vi "datalog.vi"(0 "object in":refnum<class "interface.lvclass">, 1 "data":string, 2 "filename":string="报文记录", 5 "error in (no error)":errorcluster) -> (14 "object out":refnum<class "interface.lvclass">, 19 "error out":errorcluster)   [LabVIEW 2016, in "interface.lvclass"]
uses:
  interface.lvclass
panel:
  out "路径":path
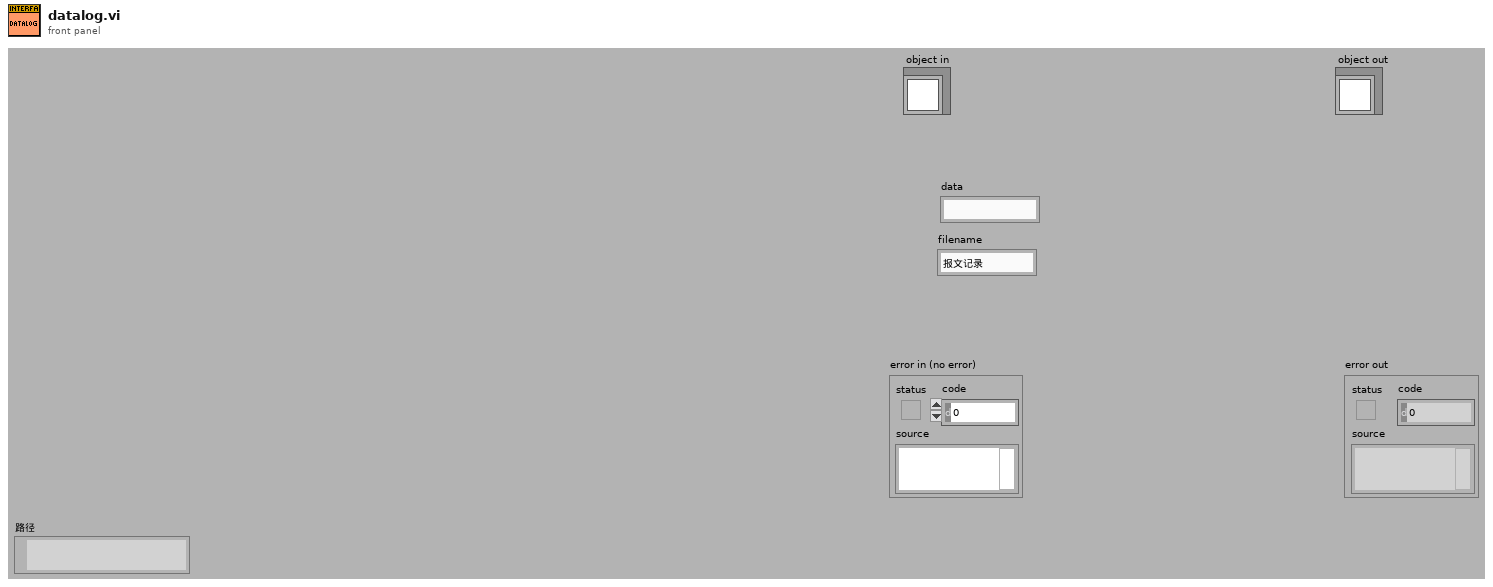
[diagram p1: front panel]
types:
  T1 = enum16{"open", "replace", "create", "open or create", "replace or create", "replace or create with confirmation"}
  T2 = typedef "LVDateTimeRec.ctl" = cluster{"秒数的小数部分":dbl, "秒":i32, "分":i32, "时":i32, "日":i32, "月":i32, "年":i32, "天数（周）":i32, "天数（年）":i32, "DST":i32}
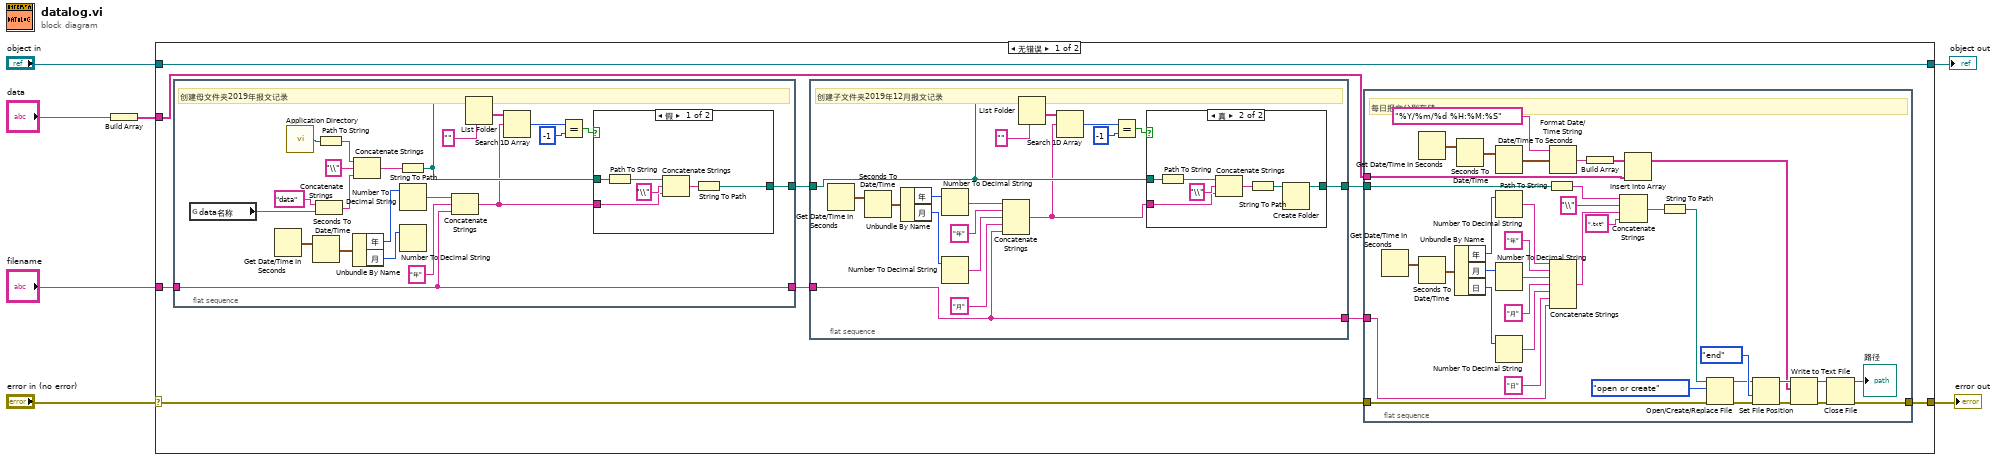
[diagram p0: block diagram]
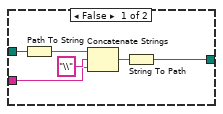
[diagram p2: hidden frame]
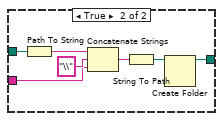
[diagram p3: hidden frame]
diagram:
  n1 = Build Array("data") -> (w1:string[])
  n2 = case shown="无错误" "error in (no error)" {
    selector: "error in (no error)" -> [w8 w121]
    tunnel: [w9 w121] -> w6
    tunnel: [w16 w120] -> w4
    tunnel: "object in" -> [w16 w120]
    tunnel: "filename" -> [w11 _]
    tunnel: w1 -> [w10 _]
    frame No Error {
      n3 = flat-sequence {
        tunnel: [w89] -> w15
        tunnel: [w86] -> w13
        tunnel: w11 -> [w86]
        frame #0 {
          # "创建母文件夹2019年报文记录"
          n4 = global read "断电保存全局.vi" "data名称"() -> (w85:string)
          n5 = Get Date/Time In Seconds() -> (seconds since 1Jan1904=w106:timestamp)
          n6 = call <vilib>:"Application Directory.vi"() -> ("Application Directory"=w94:path)
          n7 = Seconds To Date/Time(time stamp (now)=w106) -> (date time rec=w105:T2)  [unwired: 1 in]
          n8 = Concatenate Strings("data" ("名称或相对路径"), w85) -> (w87:string)
          n9 = Path To String(path=w94) -> (string=w97:string)
          n10 = Unbundle By Name(w105) -> ("年"=w104:i32, "月"=w103:i32)
          n11 = Concatenate Strings(w97, "\\" ("字符串"), w87) -> (w95:string)
          n12 = String To Path(string=w95) -> (path=w93:path)
          n13 = Number To Decimal String(number=w104) -> (decimal integer string=w91:string)  [unwired: 1 in]
          n14 = Number To Decimal String(number=w103) -> ()  [unwired: 1 in, 1 out]
          n15 = Concatenate Strings(w91, "年" ("字符串"), w86) -> (w90:string)
          n16 = List Folder(path=w93, pattern="" ("类型")) -> (folder names=w98:string[])  [unwired: 2 in, 3 out]
          n17 = Search 1D Array(1D array=w98, element=w90) -> (index of element=w102:i32)  [unwired: 1 in]
          n18 = Equal?(x=w102, y=-1) -> (x = y?=w100:bool)
          n19 = case shown="假" w100 {
            tunnel: w93 -> [w110 w118]
            tunnel: w90 -> [w109 w115]
            tunnel: [w108 w119] -> w89
            frame False {
              n20 = Path To String(path=w110) -> (string=w112:string)
              n21 = Concatenate Strings(w112, "\\" ("字符串"), w109) -> (w107:string)
              n22 = String To Path(string=w107) -> (path=w108:path)
            }
            frame True {
              n23 = Path To String(path=w118) -> (string=w117:string)
              n24 = Concatenate Strings(w117, "\\" ("字符串"), w115) -> (w113:string)
              n25 = String To Path(string=w113) -> (path=w114:path)
              n26 = Create Folder(path (use dialog)=w114) -> (created path=w119:path)  [unwired: 2 in, 2 out]
            }
          }
        }
      }
      n27 = flat-sequence {
        tunnel: w15 -> [w58]
        tunnel: [w56] -> w14
        tunnel: w13 -> [w55]
        tunnel: [w55] -> w12
        frame #0 {
          # "创建子文件夹2019年12月报文记录"
          n28 = Get Date/Time In Seconds() -> (seconds since 1Jan1904=w61:timestamp)
          n29 = Seconds To Date/Time(time stamp (now)=w61) -> (date time rec=w62:T2)  [unwired: 1 in]
          n30 = Unbundle By Name(w62) -> ("年"=w63:i32, "月"=w64:i32)
          n31 = Number To Decimal String(number=w63) -> (decimal integer string=w66:string)  [unwired: 1 in]
          n32 = Number To Decimal String(number=w64) -> (decimal integer string=w60:string)  [unwired: 1 in]
          n33 = Concatenate Strings(w66, "年" ("字符串"), w60, "月" ("字符串"), w55) -> (w57:string)
          n34 = List Folder(path=w58, pattern="" ("类型")) -> (folder names=w71:string[])  [unwired: 2 in, 3 out]
          n35 = Search 1D Array(1D array=w71, element=w57) -> (index of element=w67:i32)  [unwired: 1 in]
          n36 = Equal?(x=w67, y=-1) -> (x = y?=w69:bool)
          n37 = case shown="真" w69 {
            tunnel: w58 -> [w74 w83]
            tunnel: w57 -> [w73 w80]
            tunnel: [w72 w84] -> w56
            frame False {
              n38 = Path To String(path=w74) -> (string=w77:string)
              n39 = Concatenate Strings(w77, "\\" ("字符串"), w73) -> (w75:string)
              n40 = String To Path(string=w75) -> (path=w72:path)
            }
            frame True {
              n41 = Path To String(path=w83) -> (string=w82:string)
              n42 = Concatenate Strings(w82, "\\" ("字符串"), w80) -> (w79:string)
              n43 = String To Path(string=w79) -> (path=w78:path)
              n44 = Create Folder(path (use dialog)=w78) -> (created path=w84:path)  [unwired: 2 in, 2 out]
            }
          }
        }
      }
      n45 = flat-sequence {
        tunnel: w14 -> [w29]
        tunnel: w12 -> [w20]
        tunnel: w10 -> [w19]
        tunnel: [w18] -> w9
        tunnel: w8 -> [w17]
        frame #0 {
          # "每日报文分别存储"
          n46 = Get Date/Time In Seconds() -> (seconds since 1Jan1904=w52:timestamp)
          n47 = Get Date/Time In Seconds() -> (seconds since 1Jan1904=w23:timestamp)
          n48 = Seconds To Date/Time(time stamp (now)=w52) -> (date time rec=w51:T2)  [unwired: 1 in]
          n49 = Unbundle By Name(w51) -> ("年"=w50:i32, "月"=w49:i32, "日"=w46:i32)
          n50 = Seconds To Date/Time(time stamp (now)=w23) -> (date time rec=w26:T2)  [unwired: 1 in]
          n51 = Date/Time To Seconds(2:w26) -> (0:w24:timestamp)  [unwired: 1 in]
          n52 = Number To Decimal String(number=w50) -> (decimal integer string=w47:string)  [unwired: 1 in]
          n53 = Number To Decimal String(number=w49) -> (decimal integer string=w53:string)  [unwired: 1 in]
          n54 = Number To Decimal String(number=w46) -> (decimal integer string=w44:string)  [unwired: 1 in]
          n55 = Path To String(path=w29) -> (string=w36:string)
          n56 = Format Date/Time String(time format string (%c)="%Y/%m/%d %H:%M:%S" ("时间格式字符串(%c)"), seconds (now)=w24) -> (date/time string=w27:string)  [unwired: 1 in]
          n57 = Concatenate Strings(w47, "年" ("字符串"), w53, "月" ("字符串"), w44, "日" ("字符串"), w20) -> (w30:string)
          n58 = Build Array(w27) -> (w22:string[])
          n59 = Concatenate Strings(w36, "\\" ("字符串"), w30, ".txt" ("字符串")) -> (w38:string)
          n60 = Insert Into Array(array=w22, new element=w19) -> (w21:string[])  [unwired: 1 in]
          n61 = String To Path(string=w38) -> (path=w34:path)
          n62 = Open/Create/Replace File(file path (use dialog)=w34, error in=w17, operation (0:open)=T1."open or create" ("操作(0:open)")) -> (refnum out=w39:refnum<file>, error out=w40:errorcluster)  [unwired: 3 in, 1 out]
          n63 = Set File Position(refnum=w39, from (0:start)=enum16{"start", "end", "current"}."end" ("自（0:起始）"), error in=w40) -> (refnum out=w41:refnum<file>, error out=w42:errorcluster)  [unwired: 1 in]
          n64 = Write to Text File(file (use dialog)=w41, text=w21, error in=w42) -> (refnum out=w33:refnum<file>, error out=w32:errorcluster)  [unwired: 1 in, 1 out]
          n65 = Close File(refnum=w33, error in=w32) -> (path=→"路径":path, error out=w18:errorcluster)
        }
      }
    }
    frame Error {
    }
  }
  "error out" <- w6
  "object out" <- w4
